vi "AutoDataToString.vi"(10 "File Path Name":string[](array[string]), 11 "Auto":T1) -> (3 "String":string)   [LabVIEW 2017]
uses:
  AutoFileDataType.ctl
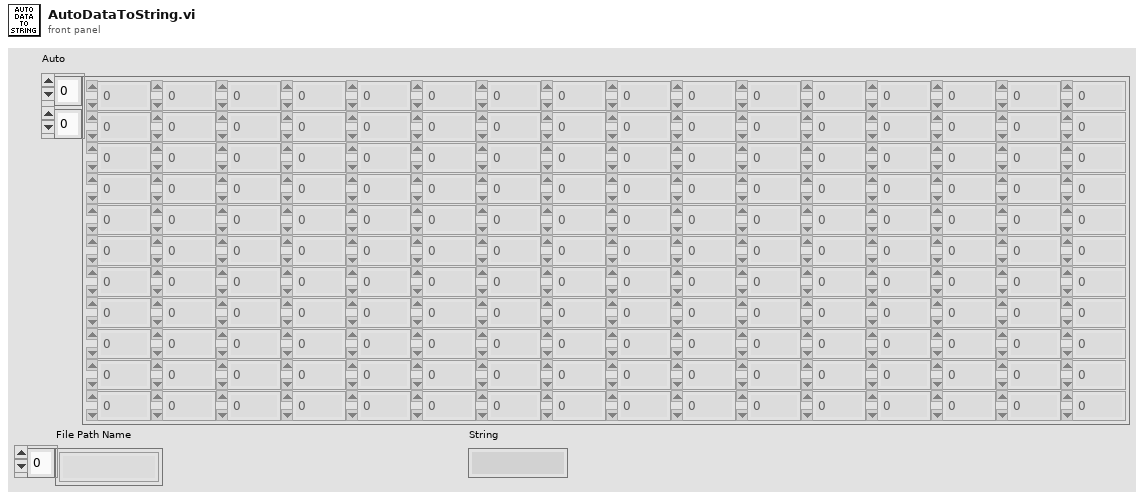
[diagram p1: front panel]
types:
  T1 = typedef "AutoFileDataType.ctl" = dbl[][]
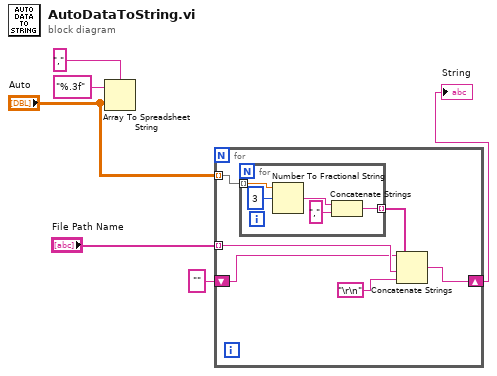
[diagram p0: block diagram]
diagram:
  n1 = Array To Spreadsheet String(delimiter (Tab)=",", array="Auto", 3:"%.3f" ("format string")) -> ()  [unwired: 1 out]
  n2 = for {
    tunnel: "Auto" -> [w12] mode=indexing
    tunnel: "File Path Name" -> [w10] mode=indexing
    shift-right: [w8] -> w1
    shift-left: "" -> [w7]
    n3 = for {
      tunnel: w12 -> [w17] mode=indexing
      tunnel: [w14] -> w11 mode=indexing
      n4 = Number To Fractional String(number=w17, precision (6)=i16 3) -> (F-format string=w16:string)  [unwired: 2 in]
      n5 = Concatenate Strings(w16, "," ("string")) -> (w14:string)
    }
    n6 = Concatenate Strings(w7, w11, w10, "\r\n") -> (w8:string)
  }
  "String" <- w1
